vi "FPGATest.vi"(8 "error in (no error)":errorcluster) -> (0 "error out":errorcluster, 3 "Telemetry":T1[](array[typedef])=[{"Address"=0, "UpdateMode"=enum."NOP", "Data"=0}, {"Address"=0, "UpdateMode"=enum."NOP", "Data"=0}, {"Address"=0, "UpdateMode"=enum."NOP", "Data"=0}, {"Address"=0, "UpdateMode"=enum."NOP", "Data"=0}, {"Address"=0, "UpdateMode"=enum."NOP", "Data"=0}, {"Address"=0, "UpdateMode"=enum."NOP", "Data"=0}, {"Address"=0, "UpdateMode"=enum."NOP", "Data"=0}, {"Address"=0, "UpdateMode"=enum."NOP", "Data"=0}, {"Address"=0, "UpdateMode"=enum."NOP", "Data"=0}, {"Address"=0, "UpdateMode"=enum."NOP", "Data"=0}, {"Address"=0, "UpdateMode"=enum."NOP", "Data"=0}, {"Address"=0, "UpdateMode"=enum."NOP", "Data"=0}, {"Address"=0, "UpdateMode"=enum."NOP", "Data"=0}, {"Address"=0, "UpdateMode"=enum."NOP", "Data"=0}, {"Address"=0, "UpdateMode"=enum."NOP", "Data"=0}, {"Address"=0, "UpdateMode"=enum."NOP", "Data"=0}, {"Address"=0, "UpdateMode"=enum."NOP", "Data"=0}, {"Address"=0, "UpdateMode"=enum."NOP", "Data"=0}, {"Address"=0, "UpdateMode"=enum."NOP", "Data"=0}, {"Address"=0, "UpdateMode"=enum."NOP", "Data"=0}, {"Address"=0, "UpdateMode"=enum."NOP", "Data"=0}, {"Address"=0, "UpdateMode"=enum."NOP", "Data"=0}, {"Address"=0, "UpdateMode"=enum."NOP", "Data"=0}, {"Address"=0, "UpdateMode"=enum."NOP", "Data"=0}, {"Address"=0, "UpdateMode"=enum."NOP", "Data"=0}, {"Address"=0, "UpdateMode"=enum."NOP", "Data"=0}, {"Address"=0, "UpdateMode"=enum."NOP", "Data"=0}, {"Address"=0, "UpdateMode"=enum."NOP", "Data"=0}, {"Address"=0, "UpdateMode"=enum."NOP", "Data"=0}, {"Address"=0, "UpdateMode"=enum."NOP", "Data"=0}, {"Address"=0, "UpdateMode"=enum."NOP", "Data"=0}, {"Address"=0, "UpdateMode"=enum."NOP", "Data"=0}, {"Address"=0, "UpdateMode"=enum."NOP", "Data"=0}, {"Address"=0, "UpdateMode"=enum."NOP", "Data"=0}, {"Address"=0, "UpdateMode"=enum."NOP", "Data"=0}, {"Address"=0, "UpdateMode"=enum."NOP", "Data"=0}, {"Address"=0, "UpdateMode"=enum."NOP", "Data"=0}, {"Address"=0, "UpdateMode"=enum."NOP", "Data"=0}, {"Address"=0, "UpdateMode"=enum."NOP", "Data"=0}, {"Address"=0, "UpdateMode"=enum."NOP", "Data"=0}, {"Address"=0, "UpdateMode"=enum."NOP", "Data"=0}, {"Address"=0, "UpdateMode"=enum."NOP", "Data"=0}, {"Address"=0, "UpdateMode"=enum."NOP", "Data"=0}, {"Address"=0, "UpdateMode"=enum."NOP", "Data"=0}, {"Address"=0, "UpdateMode"=enum."NOP", "Data"=0}, {"Address"=0, "UpdateMode"=enum."NOP", "Data"=0}, {"Address"=0, "UpdateMode"=enum."NOP", "Data"=0}, {"Address"=0, "UpdateMode"=enum."NOP", "Data"=0}, {"Address"=0, "UpdateMode"=enum."NOP", "Data"=0}, {"Address"=0, "UpdateMode"=enum."NOP", "Data"=0}, {"Address"=0, "UpdateMode"=enum."NOP", "Data"=0}, {"Address"=0, "UpdateMode"=enum."NOP", "Data"=0}, {"Address"=0, "UpdateMode"=enum."NOP", "Data"=0}, {"Address"=0, "UpdateMode"=enum."NOP", "Data"=0}, {"Address"=0, "UpdateMode"=enum."NOP", "Data"=0}, {"Address"=0, "UpdateMode"=enum."NOP", "Data"=0}, {"Address"=0, "UpdateMode"=enum."NOP", "Data"=0}, {"Address"=0, "UpdateMode"=enum."NOP", "Data"=0}, {"Address"=0, "UpdateMode"=enum."NOP", "Data"=0}, {"Address"=0, "UpdateMode"=enum."NOP", "Data"=0}, {"Address"=0, "UpdateMode"=enum."NOP", "Data"=0}, {"Address"=0, "UpdateMode"=enum."NOP", "Data"=0}, {"Address"=0, "UpdateMode"=enum."NOP", "Data"=0}, {"Address"=0, "UpdateMode"=enum."NOP", "Data"=0}, {"Address"=0, "UpdateMode"=enum."NOP", "Data"=0}, {"Address"=0, "UpdateMode"=enum."NOP", "Data"=0}, {"Address"=0, "UpdateMode"=enum."NOP", "Data"=0}, {"Address"=0, "UpdateMode"=enum."NOP", "Data"=0}, {"Address"=0, "UpdateMode"=enum."NOP", "Data"=0}, {"Address"=0, "UpdateMode"=enum."NOP", "Data"=0}, {"Address"=0, "UpdateMode"=enum."NOP", "Data"=0}, {"Address"=0, "UpdateMode"=enum."NOP", "Data"=0}, {"Address"=0, "UpdateMode"=enum."NOP", "Data"=0}, {"Address"=0, "UpdateMode"=enum."NOP", "Data"=0}, {"Address"=0, "UpdateMode"=enum."NOP", "Data"=0}, {"Address"=0, "UpdateMode"=enum."NOP", "Data"=0}, {"Address"=0, "UpdateMode"=enum."NOP", "Data"=0}, {"Address"=0, "UpdateMode"=enum."NOP", "Data"=0}, {"Address"=0, "UpdateMode"=enum."NOP", "Data"=0}, {"Address"=0, "UpdateMode"=enum."NOP", "Data"=0}, {"Address"=0, "UpdateMode"=enum."NOP", "Data"=0}, {"Address"=0, "UpdateMode"=enum."NOP", "Data"=0}, {"Address"=0, "UpdateMode"=enum."NOP", "Data"=0}, {"Address"=0, "UpdateMode"=enum."NOP", "Data"=0}, {"Address"=0, "UpdateMode"=enum."NOP", "Data"=0}, {"Address"=0, "UpdateMode"=enum."NOP", "Data"=0}, {"Address"=0, "UpdateMode"=enum."NOP", "Data"=0}, {"Address"=0, "UpdateMode"=enum."NOP", "Data"=0}, {"Address"=0, "UpdateMode"=enum."NOP", "Data"=0}, {"Address"=0, "UpdateMode"=enum."NOP", "Data"=0}, {"Address"=0, "UpdateMode"=enum."NOP", "Data"=0}, {"Address"=0, "UpdateMode"=enum."NOP", "Data"=0}, {"Address"=0, "UpdateMode"=enum."NOP", "Data"=0}, {"Address"=0, "UpdateMode"=enum."NOP", "Data"=0}, {"Address"=0, "UpdateMode"=enum."NOP", "Data"=0}, {"Address"=0, "UpdateMode"=enum."NOP", "Data"=0}, {"Address"=0, "UpdateMode"=enum."NOP", "Data"=0}, {"Address"=0, "UpdateMode"=enum."NOP", "Data"=0}, {"Address"=0, "UpdateMode"=enum."NOP", "Data"=0}, {"Address"=0, "UpdateMode"=enum."NOP", "Data"=0}])   [LabVIEW 2018]
uses:
  ts_m1m3supportFPGA/src/Common_FPGA_HealthAndStatus/DataTypes/HealthAndStatusUpdate.ctl
  ts_m1m3supportFPGA/src/Common_FPGA_HealthAndStatus/DataTypes/HealthAndStatusUpdateMode.ctl
  TestMPU.lvclass
  src/MPU.lvclass
  <vilib>/rvi/Emulation/niFpgaGetClockAttributes.vi
  <vilib>/rvi/Emulation/niFpgaSctlEmulationGetInTimedLoop.vi
  <vilib>/rvi/Emulation/niFpgaEmulationReportErrorSimple.vi
  <vilib>/rvi/Emulation/niFpgaProcessEmulError.vi
  <vilib>/rvi/interface/RandomDataEmulation/niFpgaRandomDataHandleErrors.vi
  <vilib>/rvi/Emulation/niFpgaEmulationIsFPGAContextNoSignature.vi
  <vilib>/rvi/errors/niFpgaSetErrorForExecOnDevCompSimple.vi
  <vilib>/rvi/eio/common/nirviEmuReportErrorAndStop.vi
  <vilib>/rvi/DataTransferAndStorage/Container/Common/niFpgaContainerGetUniqueNameForEmu.vi
  <vilib>/rvi/FIFO/Fifo_Resource/nirvififoEmulationSetSize.vi
  <vilib>/rvi/FIFO/Fifo_Resource/nirviFifoEmulationQueueMgr.vi
  <instcachedir>/0/nirviFifoEmulationQueueMgr_E5CAEC123FF24DC58D834DCA3CDAA9B5.lvgen/nirviFifoEmulationQueueMgr_E5CAEC123FF24DC58D834DCA3CDAA9B5_001.vi
  <vilib>/rvi/FIFO/Fifo_Resource/nirvififoEmulationDetermineInputValidOut.vi
  <vilib>/rvi/FIFO/Fifo_Resource/nirvififoEmulationCreateLock.vi
  <vilib>/rvi/FIFO/Fifo_Resource/nirvififoEmulationObtainLock.vi
  <vilib>/rvi/FIFO/Fifo_Resource/nirvififoEmulationReleaseLock.vi
  <vilib>/rvi/occurrence/nirviWaitOnOccurrenceBase.vi
  <vilib>/rvi/errors/nirviReportUnexpectedCaseInternalError.vi
  <vilib>/rvi/errors/nirviReportUnexpectedCaseInternalError (U32).vi
  <vilib>/rvi/Emulation/niFpgaCriticalErrorInLSC.vi
  <vilib>/Utility/error.llb/Clear Errors.vi
  <vilib>/rvi/DataTransferAndStorage/Container/Common/niFpgaContainerSetEmuInfo.vi
  <vilib>/rvi/DataTransferAndStorage/Container/Common/niFpgaContainerExecOnDevCompGetState.vi
  <instcachedir>/0/nirviFifoEmulationQueueMgr_E5CAEC123FF24DC58D834DCA3CDAA9B5.lvgen/nirviFifoEmulationQueueMgr_E5CAEC123FF24DC58D834DCA3CDAA9B5_022.vi
  <vilib>/rvi/DataTransferAndStorage/Container/XNode/niFpgaContainer.xnode
  <vilib>/rvi/interface/RandomDataEmulation/nirviRandomDataFpgaReadWriteTemplate.vi
  <vilib>/rvi/FIFO/Fifo_Resource/nirvififoEmulationWrite.vi
  <vilib>/rvi/FIFO/Fifo_Resource/nirvififoEmulationRead.vi
  <vilib>/rvi/LocalResourceManager/LocalResourceManager.xnode
  <vilib>/rvi/FIFO/Fifo_Resource/niFpgaFifoEmulationRefIn.vi
  ts_m1m3supportFPGA/src/Common_FPGA_HealthAndStatus/FPGAHealthAndStatus.lvlib
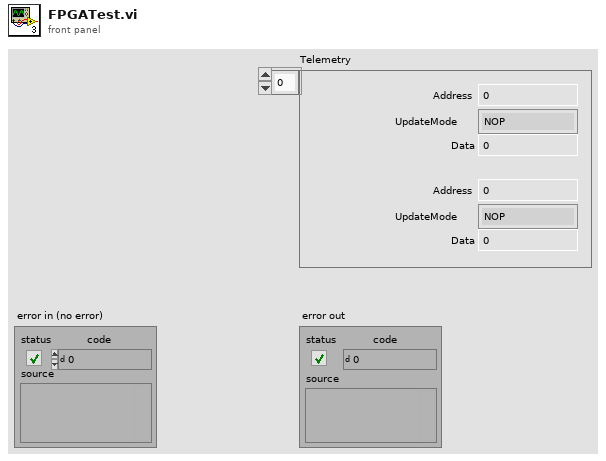
[diagram p1: front panel]
types:
  T1 = typedef "FPGAHealthAndStatus.lvlib/HealthAndStatusUpdate.ctl" = cluster{"Address":u32, "UpdateMode":T2, "Data":u64}
  T2 = typedef "FPGAHealthAndStatus.lvlib/HealthAndStatusUpdateMode.ctl" = enum8{"NOP", "Set", "Add", "Subtract", "Or", "Not And"}
  T3 = cluster{"Address":u32, "UpdateMode":enum8{"NOP", "Set", "Add", "Subtract", "Or", "Not And"}, "Data":u64}
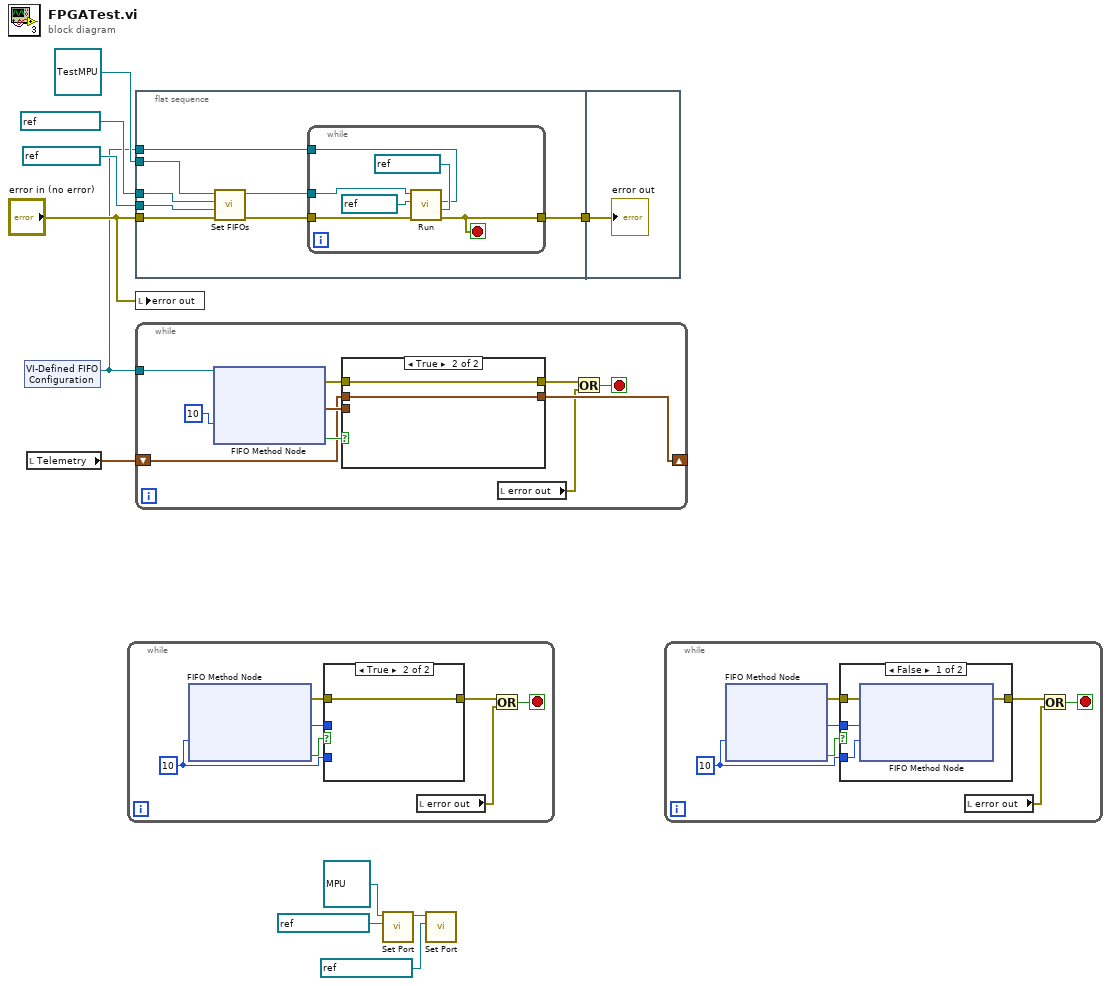
[diagram p0: block diagram]
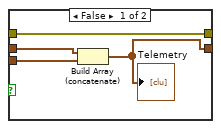
[diagram p2: hidden frame]
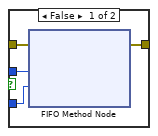
[diagram p4: hidden frame]
diagram:
  n1 = xnode "VI-Defined FIFO Configuration"() -> ("FIFO Out"=w2:refnum<k21>)
  n2 = local read "Telemetry"() -> (w1:T1[])
  n3 = while {
    stop <- w15 stop-if-true
    w17 = 10 ("Timeout")
    n4 = xnode ("FIFO Method Node")("Timeout"=w17) -> ("Element"=w18:i16, "Timed Out?"=w12:bool, "error out"=w16:errorcluster)  [unwired: 2 in, 1 out]
    n5 = case shown="True" w12 {
      tunnel: w18 -> [w22 _]
      tunnel: w17 -> [w21 _]
      tunnel: w16 -> [w20 w23]
      tunnel: [w19 w23] -> w14
      frame False {
        n6 = xnode ("FIFO Method Node")("Element"=w22, "Timeout"=w21, "error in (no error)"=w20) -> ("error out"=w19:errorcluster)  [unwired: 1 in, 2 out]
      }
      frame True {
      }
    }
    n7 = local read "error out"() -> (w13:errorcluster)
    n8 = Or(x=w14, y=w13) -> (x .or. y?=w15:bool)
  }
  n9 = flat-sequence {
    tunnel: "error in (no error)" -> [w31]
    tunnel: refnum<class "TestMPU.lvclass"> refnum ("TestMPU.lvclass") -> [w29]
    tunnel: refnum<k21> "WriteFIFO" ("Input") -> [w27]
    tunnel: refnum<k21> "ReadFIFO" ("Output") -> [w26]
    tunnel: [w25] -> w4
    tunnel: w2 -> [w24]
    tunnel: w4 -> [w38]
    frame #0 {
      n10 = call-dynamic "Set FIFOs.vi"("error in (no error)"=w31, "Output"=w26, "Input"=w27, "TestMPU in"=w29) -> ("error out"=w30:errorcluster, "TestMPU out"=w28:refnum<class "TestMPU.lvclass">)  [unwired: 6 in]
      n11 = while {
        tunnel: [w34] -> w25
        tunnel: w30 -> [w35]
        tunnel: w28 -> [w37]
        tunnel: w24 -> [w32]
        stop <- w34 stop-if-true
        n12 = call-dynamic "Run.vi"("DebugOut"=refnum<k21> "Output", "Telemetry"=w32, "error in (no error)"=w35, "Command FIFO"=refnum<k21> "Input" ("FIFO"), "MPU in"=w37) -> ("error out"=w34:errorcluster)  [unwired: 4 in, 1 out]
      }
    }
    frame #1 {
      "error out" <- w38
    }
  }
  n13 = local write "error out"("error in (no error)") -> ()
  n14 = while {
    tunnel: w2 -> [w42]
    shift-right: [w40] -> _
    shift-left: w1 -> [w41]
    stop <- w45 stop-if-true
    n15 = xnode ("FIFO Method Node")("Timeout"=10, "FIFO In"=w42) -> ("Element"=w48:T3, "Timed Out?"=w43:bool, "error out"=w46:errorcluster)  [unwired: 1 in, 1 out]
    n16 = case shown="True" w43 {
      tunnel: w48 -> [w49 _]
      tunnel: w46 -> [w52 w54]
      tunnel: [w52 w54] -> w44
      tunnel: w41 -> [w51 w53]
      tunnel: [w50 w53] -> w40
      frame False {
        n17 = Build Array (concatenate)(w51, w49) -> (w50:T1[])
        "Telemetry" <- w50
      }
      frame True {
      }
    }
    n18 = local read "error out"() -> (w39:errorcluster)
    n19 = Or(x=w44, y=w39) -> (x .or. y?=w45:bool)
  }
  n20 = call-dynamic "Set Port.vi"("Port"=refnum<k21> "Mod1\\Port1", "MPU in"=refnum<class "MPU.lvclass"> refnum ("Modbus_Processing_Unit.lvlib:MPU.lvclass")) -> ("MPU out"=w8:refnum<class "MPU.lvclass">)  [unwired: 8 in, 1 out]
  n21 = call-dynamic "Set Port.vi"("Port"=refnum<k21> "Mod2\\Port1", "MPU in"=w8) -> ()  [unwired: 8 in, 2 out]
  n22 = while {
    stop <- w57 stop-if-true
    w60 = 10 ("Timeout")
    n23 = xnode ("FIFO Method Node")("Timeout"=w60) -> ("Element"=w61:u8, "Timed Out?"=w55:bool, "error out"=w59:errorcluster)  [unwired: 2 in, 1 out]
    n24 = case shown="False" w55 {
      tunnel: w61 -> [w65 _]
      tunnel: w60 -> [w64 _]
      tunnel: w59 -> [w63 w66]
      tunnel: [w62 w66] -> w58
      frame False {
        n25 = xnode ("FIFO Method Node")("Element"=w65, "Timeout"=w64, "error in (no error)"=w63) -> ("error out"=w62:errorcluster)  [unwired: 1 in, 2 out]
      }
      frame True {
      }
    }
    n26 = local read "error out"() -> (w56:errorcluster)
    n27 = Or(x=w58, y=w56) -> (x .or. y?=w57:bool)
  }
